vi "OutsideHandle.vi"(7 "Mode":enum16{"Open", "Read", "Write", "Close"}(ring), 8 "error in (no error)":errorcluster, 10 "data in":string, 11 "Cluster":cluster{"Machine":string, "Port":u16}={"Machine"="localhost", "Port"=6342}) -> (0 "error out":errorcluster, 2 "data out":string)   [LabVIEW 2011]
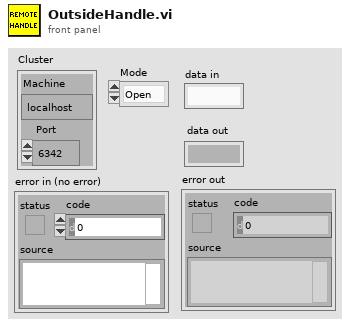
[diagram p1: front panel]
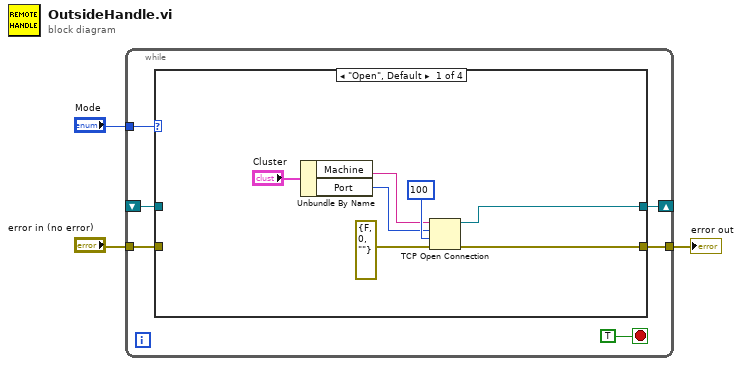
[diagram p0: block diagram]
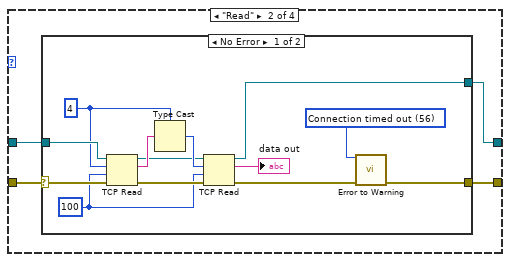
[diagram p2: hidden frame]
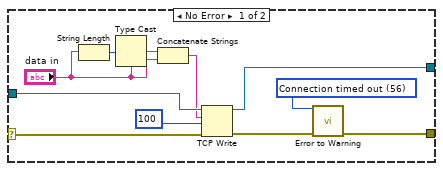
[diagram p5: hidden frame]
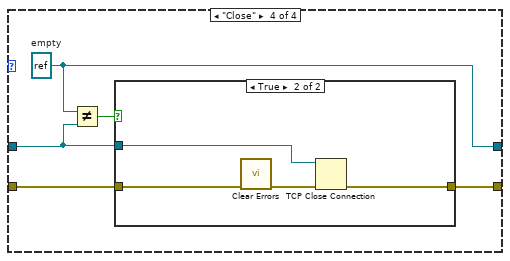
[diagram p6: hidden frame]
diagram:
  n1 = while {
    shift-right: [w9] -> _
    shift-left: _ -> [w6]
    tunnel: "Mode" -> [w5]
    tunnel: "error in (no error)" -> [w7]
    tunnel: [w8] -> w1
    stop <- TRUE stop-if-true
    n2 = case shown="\"Open\", Default" w5 {
      tunnel: [w15 w19 w36 w53] -> w9
      tunnel: [w13 w17 w38 w57] -> w8
      tunnel: w7 -> [_ w18 w37 w56]
      tunnel: w6 -> [_ w20 w39 w54]
      frame "Open", Default {
        n3 = Unbundle By Name("Cluster") -> ("Machine"=w11:string, "Port"=w10:u16)
        n4 = TCP Open Connection(address=w11, remote port or service name=w10, timeout ms (60000)=100, error in (no error)=errorcluster {"status"=FALSE, "code"=0, "source"=""} ("error constant")) -> (connection ID=w15:refnum<k5>, error out=w13:errorcluster)  [unwired: 1 out]
      }
      frame "Read" {
        n5 = case shown="No Error" w18 {
          selector: w18 -> [w32 w34]
          tunnel: w20 -> [w33 w35]
          tunnel: [w22 w35] -> w19
          tunnel: [w23 w34] -> w17
          frame No Error {
            w21 = 56 items=["No Error", "Argument Error", "Memory Full", "Out of Zone", "End of File", "File Already Open", "Generic File IO Error", "File Not Found", "File Permission Error", "Disk Full", "Duplicate Path", "Too Many Files Open", "Not Enabled", "Resource File Not Found", "Cannot Add Resource", "Resource Not Found", "Image Not Found", "Image Memory Error", "Pen Does Not Exist", "Config Bad Type", "Config Token Not Found", "Config Parse Error", "Config Memory Error", "Bad External Code Format", "Bad External Code Offset", "External Code Not Present", "Null Window", "Destroy Window Mixup", "Null Menu", "Print Aborted", "Bad Print Record", "Print Driver Error", "Windows Error During Print", "Memory Error During Print", "Print Dialog Error", "Generic Print Error", "Invalid Device Refnum", "Device Not Found", "Device Parameter Error", "Device Unit Error", "Can't Open Device", "Device Call Aborted", "Generic Error", "Cancelled By User", "Object ID Too Low", "Object ID Too High", "Object Not In Heap", "Unknown Heap", "Bad DefProc ID", "DefProc Not In Table", "Message Out Of Range", "Null Method", "Unknown Message", "Manager Call Not Supported", "Bad address", "Connection In progress", "Connection timed out", "Connection is already in progress", "Network attribute not supported", "Network error", "Address in use", "System out of memory", "Connection aborted", "Connection refused", "Connection is not connected", "Connection is already connected", "Connection closed", "Initialize error (interapplication manager)", "Bad occurrence", "Wait on unbound occurrence handler", "Occurrence queue overflow", "Bad path", "Semaphore not signaled", "Unrecognized type (interapplication manager)"] ("1st Error to Convert")
            w28 = 100
            w25 = 4 ("bytes to read")
            n6 = TCP Read(connection ID=w33, bytes to read=w25, error in (no error)=w32, 9:w28) -> (connection ID out=w26:refnum<k5>, data out=w27:string, error out=w29:errorcluster)  [unwired: 1 out]
            n7 = Type Cast(type=w25, x=w27) -> (*(type *) &x=w30:i32)
            n8 = TCP Read(connection ID=w26, bytes to read=w30, error in (no error)=w29, 9:w28) -> (connection ID out=w22:refnum<k5>, data out=→"data out":string, error out=w24:errorcluster)  [unwired: 1 out]
            n9 = call <vilib>:"Error to Warning.vi"("1st Error to Convert"=w21, "error in"=w24) -> ("warning out"=w23:errorcluster)  [unwired: 3 in, 10 out]
          }
          frame Error {
          }
        }
      }
      frame "Write" {
        n10 = case shown="Error" w37 {
          selector: w37 -> [w47 w51]
          tunnel: w39 -> [w50 w52]
          tunnel: [w42 w52] -> w36
          tunnel: [w48 w51] -> w38
          frame No Error {
            w41 = 56 items=["No Error", "Argument Error", "Memory Full", "Out of Zone", "End of File", "File Already Open", "Generic File IO Error", "File Not Found", "File Permission Error", "Disk Full", "Duplicate Path", "Too Many Files Open", "Not Enabled", "Resource File Not Found", "Cannot Add Resource", "Resource Not Found", "Image Not Found", "Image Memory Error", "Pen Does Not Exist", "Config Bad Type", "Config Token Not Found", "Config Parse Error", "Config Memory Error", "Bad External Code Format", "Bad External Code Offset", "External Code Not Present", "Null Window", "Destroy Window Mixup", "Null Menu", "Print Aborted", "Bad Print Record", "Print Driver Error", "Windows Error During Print", "Memory Error During Print", "Print Dialog Error", "Generic Print Error", "Invalid Device Refnum", "Device Not Found", "Device Parameter Error", "Device Unit Error", "Can't Open Device", "Device Call Aborted", "Generic Error", "Cancelled By User", "Object ID Too Low", "Object ID Too High", "Object Not In Heap", "Unknown Heap", "Bad DefProc ID", "DefProc Not In Table", "Message Out Of Range", "Null Method", "Unknown Message", "Manager Call Not Supported", "Bad address", "Connection In progress", "Connection timed out", "Connection is already in progress", "Network attribute not supported", "Network error", "Address in use", "System out of memory", "Connection aborted", "Connection refused", "Connection is not connected", "Connection is already connected", "Connection closed", "Initialize error (interapplication manager)", "Bad occurrence", "Wait on unbound occurrence handler", "Occurrence queue overflow", "Bad path", "Semaphore not signaled", "Unrecognized type (interapplication manager)"] ("1st Error to Convert")
            n11 = String Length(string="data in") -> (length=w45:i32)
            n12 = Type Cast(type="data in", x=w45) -> (*(type *) &x=w46:string)
            n13 = Concatenate Strings(w46, "data in") -> (w44:string)
            n14 = TCP Write(connection ID=w50, data in=w44, error in (no error)=w47, 9:100 ("timeout ms (25000)")) -> (connection ID out=w42:refnum<k5>, error out=w43:errorcluster)  [unwired: 1 out]
            n15 = call <vilib>:"Error to Warning.vi"("1st Error to Convert"=w41, "error in"=w43) -> ("warning out"=w48:errorcluster)  [unwired: 3 in, 10 out]
          }
          frame Error {
          }
        }
      }
      frame "Close" {
        w53 = refnum<k5> refnum  # empty
        n16 = Not Equal?(x=w53, y=w54) -> (x != y?=w55:bool)
        n17 = case shown="True" w55 {
          tunnel: [w58 w62] -> w57
          tunnel: w56 -> [w58 w61]
          tunnel: w54 -> [_ w59]
          frame False {
          }
          frame True {
            n18 = call <vilib>:"Clear Errors.vi"("error in (no error)"=w61) -> ("error out"=w60:errorcluster)  [unwired: 6 in]
            n19 = TCP Close Connection(connection ID=w59, error in (no error)=w60) -> (error out=w62:errorcluster)  [unwired: 2 out]
          }
        }
      }
    }
  }
  "error out" <- w1
